vi "Builder.Initialize Intermediate Buffers.vi"(8 "error in (no error)":errorcluster, 11 "Builder in":refnum<class "Builder.lvclass">) -> (0 "error out":errorcluster, 1 "VS Channels Buffer":dbl[](array[numeric]), 2 "Data Type Buffers":T1, 3 "Builder out":refnum<class "Builder.lvclass">)   [LabVIEW 2016, in "DSF.Engine.lvlib" / "Builder.lvclass"]
uses:
  Builder.lvclass
  DSF.Engine.Typedefs.Type Buffers.ctl
  Builder.lvclass/Builder.ctl
  Cache/DSF.Engine.Memory.Cache.Framework.lvclass
  DSF.Engine.lvlib
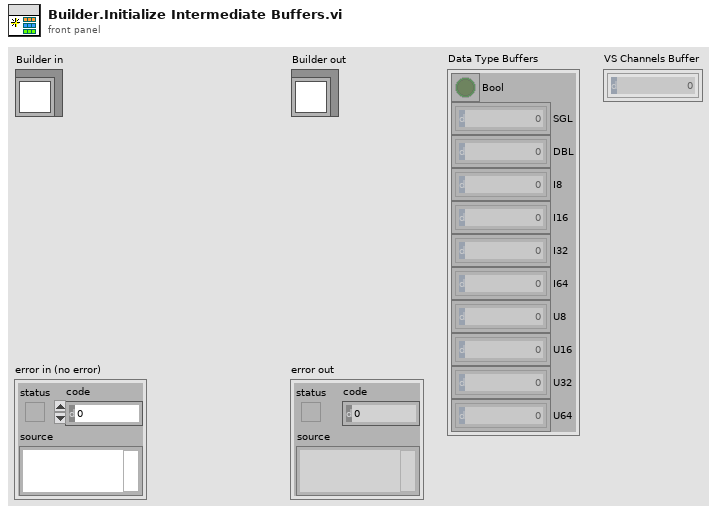
[diagram p1: front panel]
types:
  T1 = typedef "DSF.Engine.lvlib/DSF.Engine.Typedefs.Type Buffers.ctl" = cluster{"Bool":bool[], "SGL":sgl[], "DBL":dbl[], "I8":i8[], "I16":i16[], "I32":i32[], "I64":i64[], "U8":u8[], "U16":u16[], "U32":u32[], "U64":u64[]}
  T2 = typedef "DSF.Shared.lvlib/DSF.Shared.Typedefs.Data Type Counts.ctl" = cluster{"Bool":u64, "SGL":u64, "DBL":u64, "I8":u64, "I16":u64, "I32":u64, "I64":u64, "U8":u64, "U16":u64, "U32":u64, "U64":u64}
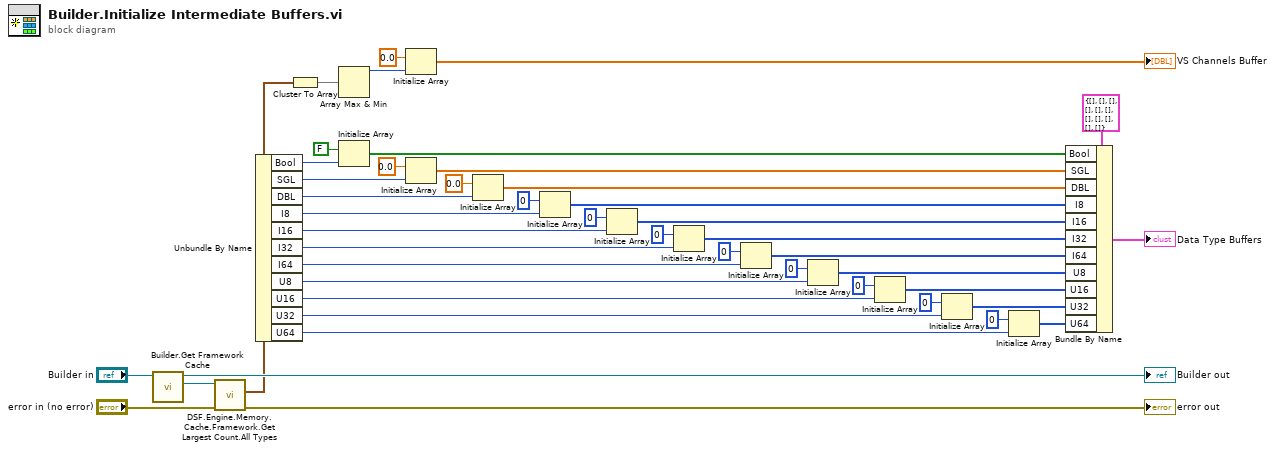
[diagram p0: block diagram]
diagram:
  n1 = call "Builder.Get Framework Cache.vi"("Builder in"="Builder in") -> ("Framework Cache"=w9:refnum<class "DSF.Engine.Memory.Cache.Framework.lvclass">, "Builder out"=→"Builder out":refnum<class "Builder.lvclass">)  [unwired: 9 in]
  n2 = call "DSF.Engine.Memory.Cache.Framework.Get Largest Count.All Types.vi"("error in (no error)"="error in (no error)", "Framework Cache in"=w9) -> ("error out"=→"error out":errorcluster, "Data Type Counts out"=w1:T2)  [unwired: 7 in, 1 out]
  n3 = Unbundle By Name(w1) -> ("Bool"=w44:u64, "SGL"=w42:u64, "DBL"=w36:u64, "I8"=w33:u64, "I16"=w25:u64, "I32"=w24:u64, "I64"=w23:u64, "U8"=w22:u64, "U16"=w21:u64, "U32"=w20:u64, "U64"=w19:u64)
  n4 = Cluster To Array(cluster=w1) -> (array=w5:u64[])
  n5 = Array Max & Min(array=w5) -> (max value=w4:u64)  [unwired: 3 out]
  n6 = Initialize Array(FALSE, w44) -> (w40:bool[])
  n7 = Initialize Array(0.0 ("element"), w4) -> (→"VS Channels Buffer":dbl[])
  n8 = Initialize Array(sgl 0.0, w42) -> (w39:sgl[])
  n9 = Initialize Array(0.0, w36) -> (w35:dbl[])
  n10 = Initialize Array(i8 0, w33) -> (w11:i8[])
  n11 = Initialize Array(i16 0, w25) -> (w12:i16[])
  n12 = Initialize Array(0, w24) -> (w13:i32[])
  n13 = Initialize Array(i64 0, w23) -> (w14:i64[])
  n14 = Initialize Array(u8 0, w22) -> (w15:u8[])
  n15 = Initialize Array(u16 0, w21) -> (w16:u16[])
  n16 = Initialize Array(u32 0, w20) -> (w17:u32[])
  n17 = Initialize Array(u64 0, w19) -> (w18:u64[])
  n18 = Bundle By Name(cluster=T1 {"Bool"=[], "SGL"=[], "DBL"=[], "I8"=[], "I16"=[], "I32"=[], "I64"=[], "U8"=[], "U16"=[], "U32"=[], "U64"=[]} ("Data Type Buffers"), "Bool"=w40, "SGL"=w39, "DBL"=w35, "I8"=w11, "I16"=w12, "I32"=w13, "I64"=w14, "U8"=w15, "U16"=w16, "U32"=w17, "U64"=w18) -> (→"Data Type Buffers":T1)
